vi "Element Events.vi"(8 "error in (no error)":errorcluster, 11 "2WayValve in":refnum<class "2WayValveV.lvclass">) -> (0 "error out":errorcluster, 2 "Controls Events":refnum<class "Control Event Registrations.lvclass">, 3 "2WayValve out":refnum<class "2WayValveV.lvclass">)   [LabVIEW 2020, in "VolatusGUIElements.lvlib" / "2WayValveV.lvclass"]
uses:
  2WayValveV.lvclass
  2WayValveV.lvclass/2WayValveV.ctl
  VolatusGUI/GUI Element/GUI Element.lvclass
  VolatusGUI/Control Event Registrations/Control Event Registrations.lvclass
  C:/dev/lv20CE/relink/lv-volatus/VolatusGUI/GUI Element/GUI Element.lvclass
  C:/dev/lv20CE/relink/lv-volatus/VolatusGUIElements/2WayValveV/2WayValveV.lvclass
  C:/dev/lv20CE/relink/lv-volatus/VolatusGUI/OnValueChangeHandler/OnValueChangeHandler.lvclass
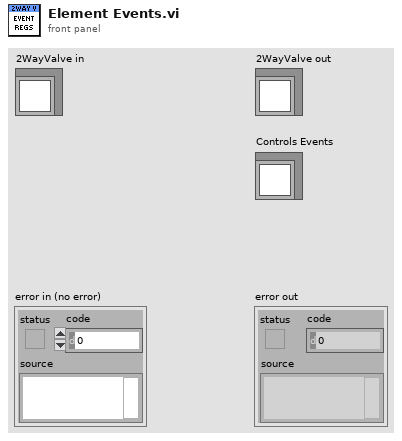
[diagram p1: front panel]
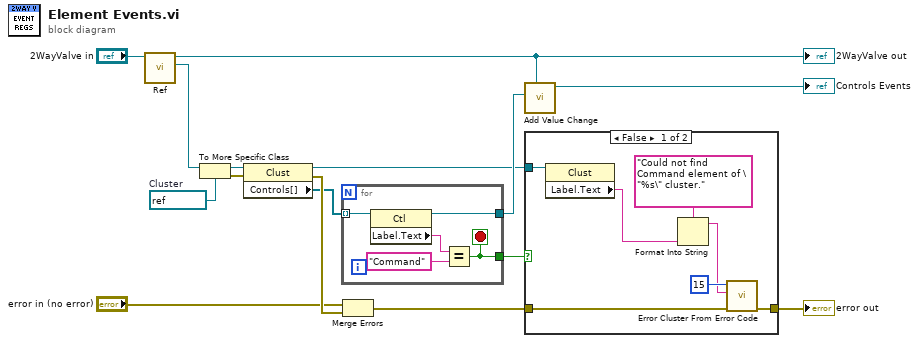
[diagram p0: block diagram]
diagram:
  w11 = refnum<vi> refnum  # Cluster
  n1 = call "Ref.vi"("GUI Element in"="2WayValve in") -> ("Ref"=w12:refnum<vi>, "GUI Element out"=w6:refnum<class "2WayValveV.lvclass">)  [unwired: 9 in]
  "2WayValve out" <- w6
  n2 = To More Specific Class(target class=w11, reference=w12) -> (specific class reference=w10:refnum<vi>, error out=w9:errorcluster)  [unwired: 1 in]
  n3 = property class="Clust"(reference=w10, error in=w9) -> (reference out=w1:refnum<vi>, error out=w15:errorcluster, "Controls[]"=w8:refnum<vi>[])
  n4 = for {
    tunnel: w8 -> [w20] mode=indexing
    tunnel: [w16] -> w4
    tunnel: [w17] -> w7
    stop <- w16 stop-if-true
    n5 = property class="Ctl"(reference=w20) -> (reference out=w17:refnum<vi>, "Label.Text"=w19:string)  [unwired: 1 in, 1 out]
    n6 = Equal?(x=w19, y="Command" ("x")) -> (x = y?=w16:bool)
  }
  n7 = Merge Errors("error in (no error)", w15) -> (w3:errorcluster)
  n8 = call "Add Value Change.vi"("Control"=w6, "CtlRef"=w7) -> ("Control Event Registrations out"=→"Controls Events":refnum<class "Control Event Registrations.lvclass">)  [unwired: 8 in, 1 out]
  n9 = case shown="False" w4 {
    tunnel: w3 -> [w26 w28]
    tunnel: [w27 w28] -> w2
    tunnel: w1 -> [w25 _]
    frame False {
      n10 = property class="Clust"(reference=w25) -> ("Label.Text"=w22:string)  [unwired: 1 in, 2 out]
      n11 = Format Into String(format string="Could not find Command element of \"%s\" cluster.", w22) -> (resulting string=w21:string)  [unwired: 2 in, 1 out]
      n12 = call <vilib>:"Error Cluster From Error Code.vi"("error in (no error)"=w26, "error message (\"\")"=w21, "error code (0)"=15) -> ("error out"=w27:errorcluster)  [unwired: 6 in]
    }
    frame True {
    }
  }
  "error out" <- w2
